vi "PhaseToSec_9215.vi"(7 "Reference Channel":u32, 8 "NumAcquisitions":u32, 9 "NumChannels":u32, 10 "Phases":dbl[](array[numeric]), 11 "Frequencies":dbl[](array[numeric])) -> (1 "Max Phase Difference Array":dbl[][](array[numeric]), 2 "Max Phase Difference":dbl, 3 "Per Channel Phase Differences":dbl[][](array[numeric]))   [LabVIEW 2018]
uses:
  <vilib>/Analysis/baseanly.llb/Mean (DBL).vi
  <vilib>/Analysis/NI_AALBase.lvlib
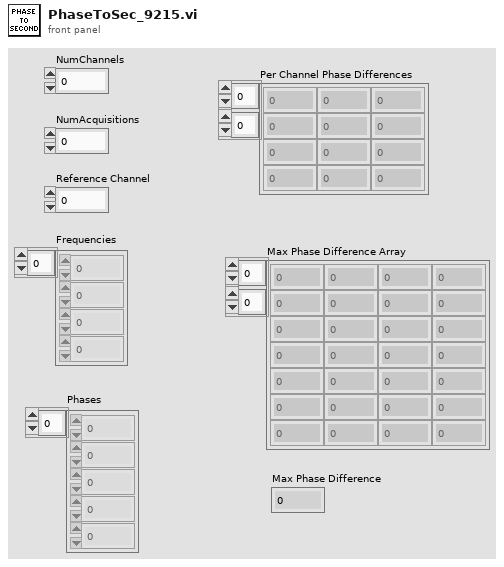
[diagram p1: front panel]
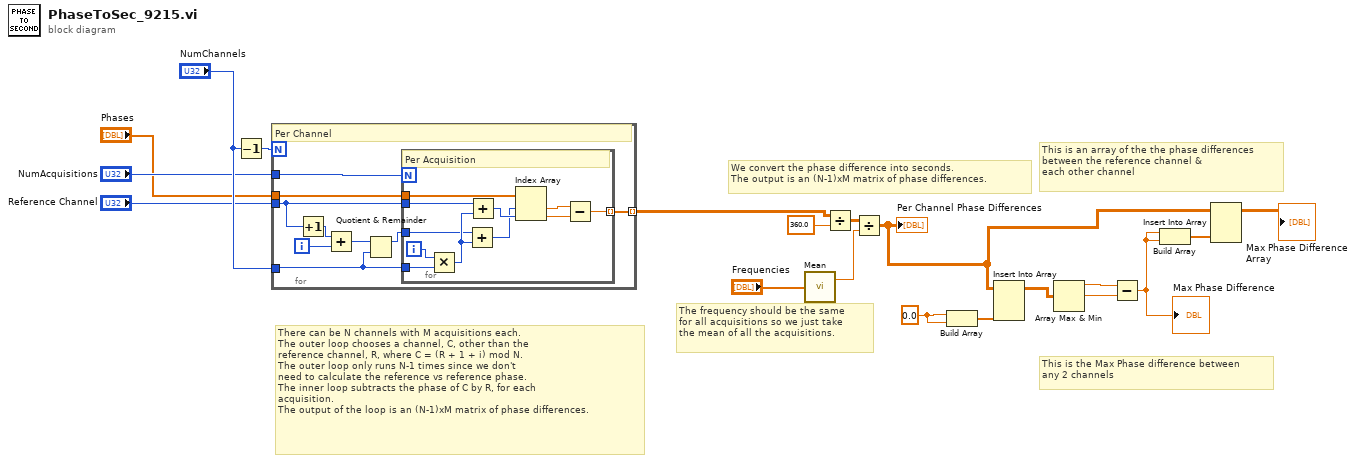
[diagram p0: block diagram]
diagram:
  w3 = 0.0 ("element")
  # "This is the Max Phase difference between\nany 2 channels"
  # "This is an array of the the phase differences\nbetween the reference channel & \neach other channel"
  # "The frequency should be the same\nfor all acquisitions so we just take\nthe mean of all the acquisitions."
  # "We convert the phase difference into seconds.\nThe output is an (N-1)xM matrix of phase differences."
  # "There can be N channels with M acquisitions each.\nThe outer loop chooses a channel, C, other than the\nreference channel, R, where C = (R + 1 + i) mod N.\nThe outer loop only runs N-1 times since we don't\nneed to calculate the reference vs reference phase.\nThe inner loop subtracts the phase of C by R, for each\nacquisition.\nThe output of the loop is an (N-1)xM matrix of phase differences."
  n1 = Decrement(x="NumChannels") -> (x-1=w18:u32)
  n2 = for {
    N: w18 -> [_]
    tunnel: "NumAcquisitions" -> [w28]
    tunnel: "NumChannels" -> [w22]
    tunnel: "Phases" -> [w27]
    tunnel: [w26] -> w10 mode=indexing
    tunnel: "Reference Channel" -> [w20]
    i -> [w24]
    # "Per Channel"
    n3 = Increment(x=w20) -> (x+1=w25:u32)
    n4 = Add(x=w25, y=w24) -> (x+y=w21:u32)
    n5 = Quotient & Remainder(x=w21, y=w22) -> (x-y*floor(x/y)=w23:u32)  [unwired: 1 out]
    n6 = for {
      N: w28 -> [_]
      tunnel: w20 -> [w39]
      tunnel: w27 -> [w37]
      tunnel: w23 -> [w29]
      tunnel: [w36] -> w26 mode=indexing
      tunnel: w22 -> [w34]
      i -> [w35]
      # "Per Acquisition"
      n7 = Multiply(x=w35, y=w34) -> (x*y=w38:u32)
      n8 = Add(x=w29, y=w38) -> (x+y=w32:u32)
      n9 = Add(x=w39, y=w38) -> (x+y=w33:u32)
      n10 = Index Array(array=w37, index #1=w32, index #2=w33) -> (element #1=w31:dbl, element #2=w30:dbl)
      n11 = Subtract(x=w31, y=w30) -> (x-y=w36:dbl)
    }
  }
  n12 = call-poly <vilib>:"Mean.vi"("X"="Frequencies") -> ("mean"=w11:dbl)  [unwired: 1 out]
  n13 = Divide(x=w10, y=360.0) -> (x/y=w13:dbl[][])
  n14 = Divide(x=w13, y=w11) -> (x/y=w1:dbl[][])
  "Per Channel Phase Differences" <- w1
  n15 = Build Array(w3, w3) -> (w4:dbl[])
  n16 = Insert Into Array(array=w1, new element=w4) -> (w2:dbl[][])  [unwired: 2 in]
  n17 = Array Max & Min(array=w2) -> (max value=w9:dbl, min value=w8:dbl)  [unwired: 2 out]
  n18 = Subtract(x=w9, y=w8) -> (x-y=w7:dbl)
  "Max Phase Difference" <- w7
  n19 = Build Array(w7, w7) -> (w6:dbl[])
  n20 = Insert Into Array(array=w1, new element=w6) -> (→"Max Phase Difference Array":dbl[][])  [unwired: 2 in]
